vi "getSubVarib.vi"(11 "Device in":string) -> (3 "data":string[][](array[string]))   [LabVIEW 2013]
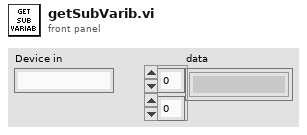
[diagram p1: front panel]
types:
  T1 = typedef "mysql_authentication.ctl" = cluster{"User":string, "Password":string, "Database":string}
  T2 = cluster{"Port":u16, "IP Address":string, "Authentication":T1}
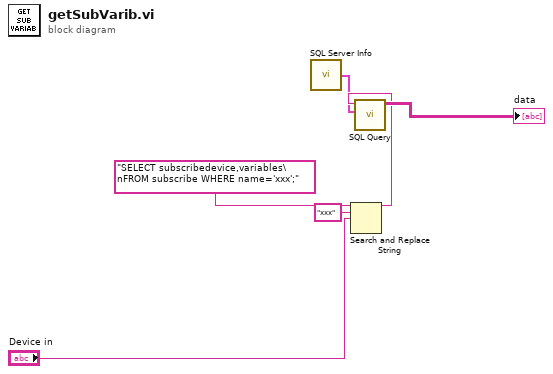
[diagram p0: block diagram]
diagram:
  n1 = call "SQL Server Info.vi"() -> ("SQL Server Info"=w1:T2)
  n2 = Search and Replace String(input string="SELECT subscribedevice,variables\nFROM subscribe WHERE name='xxx';", search string="xxx", replace string="Device in") -> (result string=w5:string)  [unwired: 5 in, 3 out]
  n3 = call "SQL Query.vi"("SQL Server Info"=w1, "Query"=w5) -> ("data"=→"data":string[][])  [unwired: 8 in, 1 out]
